vi "GET_PRODUCT_ID.vi"(11 "PRODFUCT_NAME":string="PRODUCT_NAME") -> (3 "PRODUCT_ID":string)   [LabVIEW 2020]
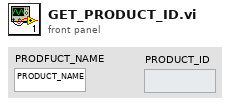
[diagram p1: front panel]
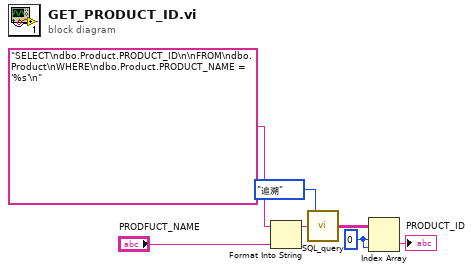
[diagram p0: block diagram]
diagram:
  w3 = 0 ("索引 (行)")
  n1 = Format Into String(format string="SELECT\ndbo.Product.PRODUCT_ID\n\nFROM\ndbo.Product\nWHERE\ndbo.Product.PRODUCT_NAME = '%s'\n" ("SQL query"), "PRODFUCT_NAME") -> (resulting string=w7:string)  [unwired: 2 in, 1 out]
  n2 = call "SQL_query.vi"("SQL query"=w7, "联机模式"=enum16{"单机", "追溯"}."追溯") -> ("data"=w4:string[][])  [unwired: 1 in, 2 out]
  n3 = Index Array(array=w4, index (row)=w3, index (col)=w3) -> (element=→"PRODUCT_ID":string)
